vi "Log.vi"(0 "object in":refnum<class "Client.lvclass">, 2 "Input":variant, 5 "error in (no error)":errorcluster) -> (14 "object out":refnum<class "Client.lvclass">, 19 "error out":errorcluster)   [LabVIEW 2024, in "Client.lvclass"]
doc: "Log given input with current data type and data method classes"
uses:
  Client.lvclass
  Support/Type Def/Requirements.ctl
  Support/Type Def/File Type.ctl
  Client.lvclass/Client.ctl
  Abstractions/DataType/DataType.lvclass
panel:
  # "Connector Pane"
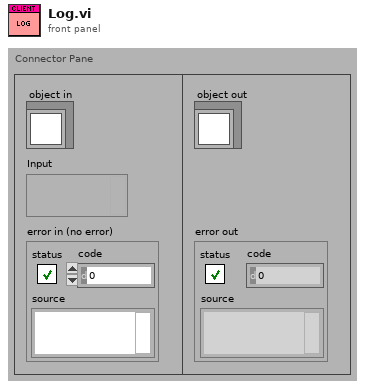
[diagram p1: front panel]
types:
  T1 = typedef "Requirements.ctl" = cluster{"From":T2, "File Handler":variant, "Input":variant}
  T2 = typedef "File Type.ctl" = enum32{"TDMS", "EXCEL"}
  T3 = typedef "Message.ctl" = cluster{"Message":string, "From":enum16{"LOGGER", "VIEWER"}, "Return":variant}
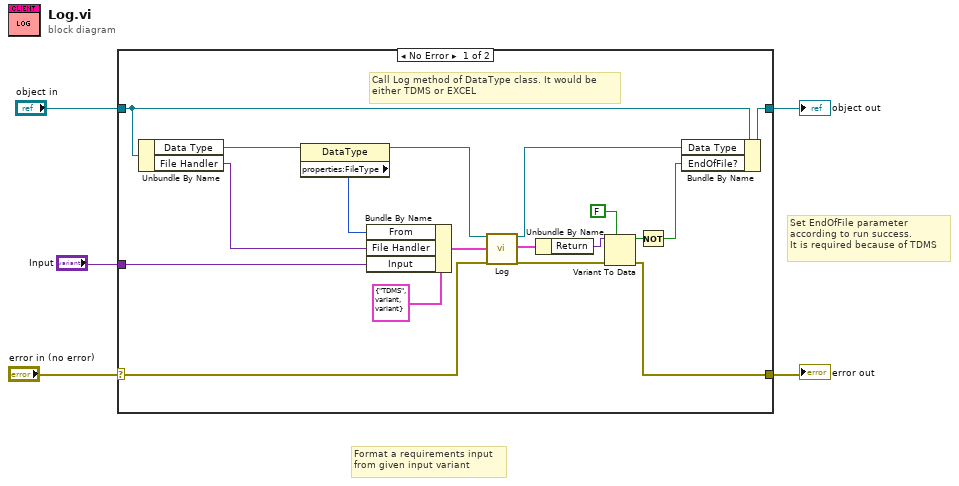
[diagram p0: block diagram]
diagram:
  # "Set EndOfFile parameter\naccording to run success.\nIt is required because of TDMS"
  # "Format a requirements input\nfrom given input variant"
  n1 = case shown="No Error" "error in (no error)" {
    selector: "error in (no error)" -> [w21 w25]
    tunnel: [w7 w25] -> w4
    tunnel: [w19 w24] -> w2
    tunnel: "object in" -> [w23 w24]
    tunnel: "Input" -> [w20 _]
    frame No Error {
      # "Call Log method of DataType class. It would be\neither TDMS or EXCEL"
      n2 = Unbundle By Name(w23) -> ("Data Type"=w22:refnum<class "DataType.lvclass">, "File Handler"=w17:variant)
      n3 = property class="DataType"(reference=w22) -> (reference out=w14:refnum<class "DataType.lvclass">, "properties:FileType"=w13:T2)  [unwired: 1 in, 1 out]
      n4 = Bundle By Name(cluster=T1 {"From"=enum."TDMS", "File Handler"=variant, "Input"=variant} ("Requirements"), "From"=w13, "File Handler"=w17, "Input"=w20) -> (w15:T1)
      n5 = call-dynamic "Log.vi"("object in"=w14, "Requirements"=w15, "error in (no error)"=w21) -> ("object out"=w18:refnum<class "DataType.lvclass">, "Message"=w12:T3, "error out"=w10:errorcluster)  [unwired: 14 in]
      n6 = Unbundle By Name(w12) -> ("Return"=w11:variant)
      n7 = Variant To Data(error in=w10, type=FALSE, Variant=w11) -> (data=w8:bool, error out=w7:errorcluster)
      n8 = Not(x=w8) -> (.not. x?=w6:bool)
      n9 = Bundle By Name(cluster=w23, "Data Type"=w18, "EndOfFile?"=w6) -> (w19:refnum<class "Client.lvclass">)
    }
    frame Error {
    }
  }
  "error out" <- w4
  "object out" <- w2
